vi "UDP - Data System (SubVI).vi"(8 "error in (no error)":errorcluster, 11 "Data":string="\u000204\u0001\u0000ÿ\u0000è\u0003\u0000\u0000\u0000\u0019\u0000\u00002\u0000\u0000\u0000\u001e\u0000\u0000\u0000\u0000\u0000@@\u0000\u0000 @Õ\u0000\u0000\u00002\u0000\u0000\u0000\u0000\u0000€?Ð\u0007\u0000\u0000K") -> (0 "error out":errorcluster, 3 "Data System":T1, 4 "Success":bool)   [LabVIEW 2019]
panel:
  in  "Data 2":string="\u0000\u0000;:\u0000ï²k7ªª5@%\u0019è?\u0000\u0000\u0000\u0000«\u0000\u0000\u0000ÈA\u0000\u0000\u0000\u0000\u000f\u0000\u0000\u0000\u0007\u0000\u0000\u0000Disp\u0000\u0000\u0000\u0000\u0000"
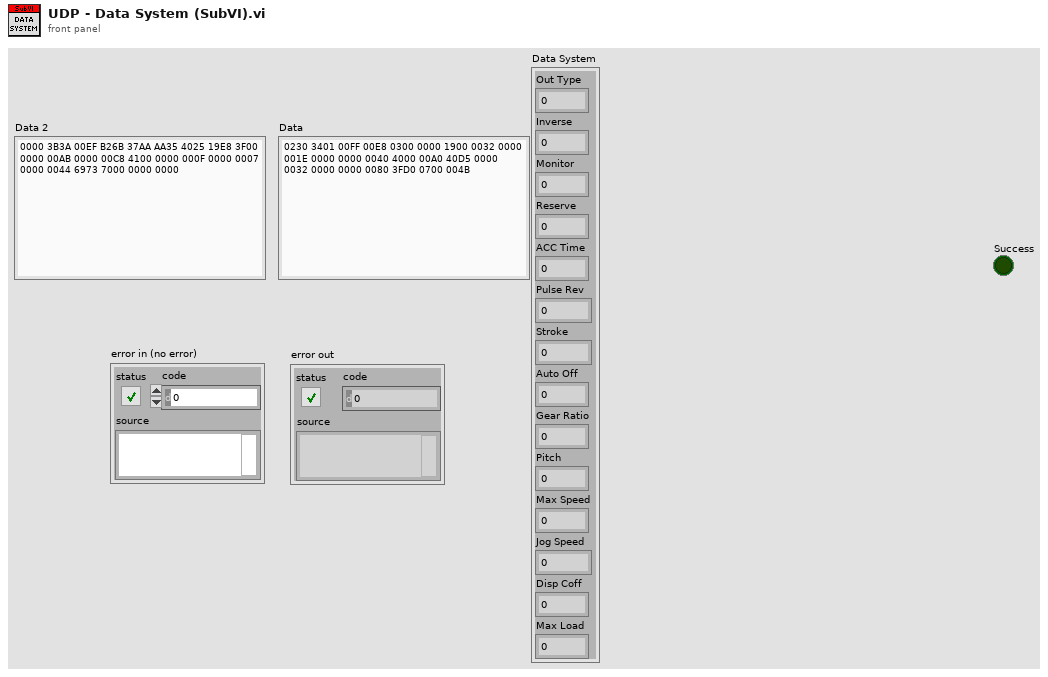
[diagram p1: front panel]
types:
  T1 = cluster{"Out Type":u8, "Inverse":u8, "Monitor":u8, "Reserve":u8, "ACC Time":u32, "Pulse Rev":u32, "Stroke":u32, "Auto Off":u32, "Gear Ratio":sgl, "Pitch":sgl, "Max Speed":u32, "Jog Speed":u32, "Disp Coff":sgl, "Max Load":u32}
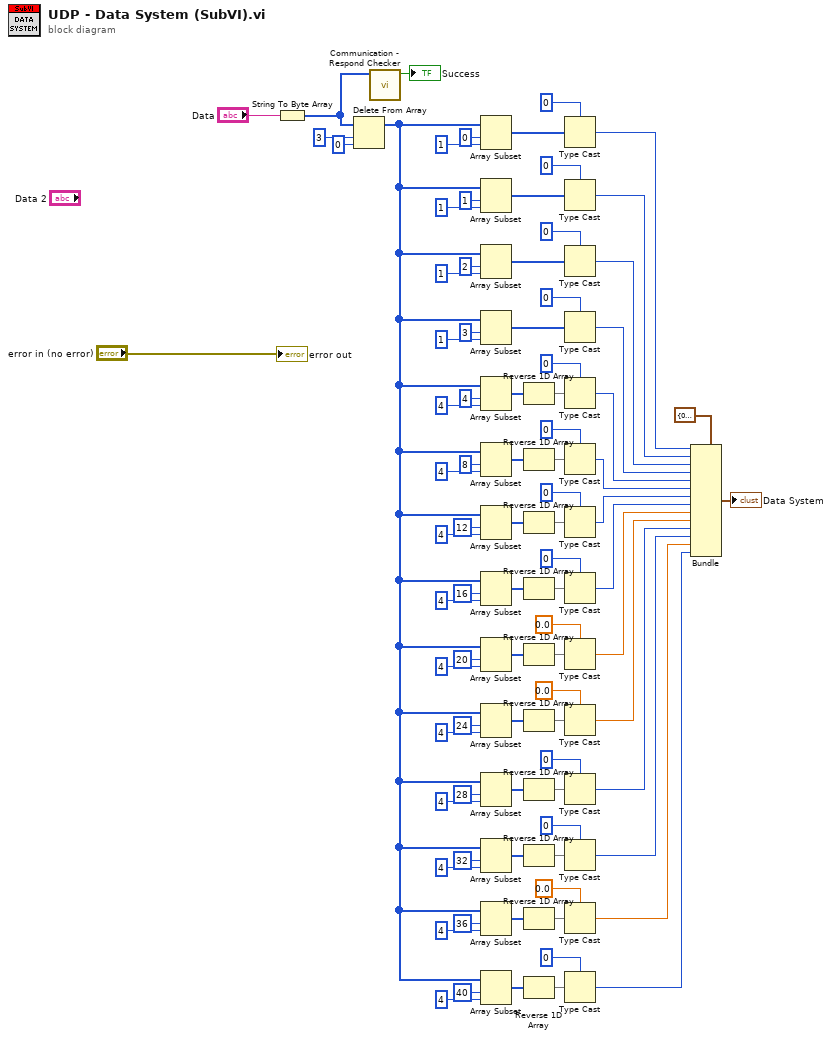
[diagram p0: block diagram]
diagram:
  n1 = String To Byte Array(string="Data") -> (unsigned byte array=w21:u8[])
  n2 = Delete From Array(array=w21, length=3, index=0) -> (array with subset deleted=w5:u8[])  [unwired: 1 out]
  n3 = call "Communication - Respond Checker.vi"("Read Data"=w21) -> ("Success"=→"Success":bool)  [unwired: 10 in]
  n4 = Array Subset(array=w5, index=0, length=1) -> (w20:u8[])
  n5 = Array Subset(array=w5, index=1, length=1) -> (w19:u8[])
  n6 = Array Subset(array=w5, index=2, length=1) -> (w18:u8[])
  n7 = Array Subset(array=w5, index=3, length=1) -> (w17:u8[])
  n8 = Array Subset(array=w5, index=4, length=4) -> (w72:u8[])
  n9 = Array Subset(array=w5, index=8, length=4) -> (w49:u8[])
  n10 = Array Subset(array=w5, index=12, length=4) -> (w54:u8[])
  n11 = Array Subset(array=w5, index=16, length=4) -> (w59:u8[])
  n12 = Array Subset(array=w5, index=20, length=4) -> (w64:u8[])
  n13 = Array Subset(array=w5, index=24, length=4) -> (w38:u8[])
  n14 = Array Subset(array=w5, index=28, length=4) -> (w44:u8[])
  n15 = Array Subset(array=w5, index=32, length=4) -> (w36:u8[])
  n16 = Array Subset(array=w5, index=36, length=4) -> (w14:u8[])
  n17 = Array Subset(array=w5, index=40, length=4) -> (w11:u8[])
  n18 = Reverse 1D Array(array=w72) -> (reversed array=w71:u8[])
  n19 = Reverse 1D Array(array=w49) -> (reversed array=w50:u8[])
  n20 = Reverse 1D Array(array=w54) -> (reversed array=w53:u8[])
  n21 = Reverse 1D Array(array=w59) -> (reversed array=w60:u8[])
  n22 = Reverse 1D Array(array=w64) -> (reversed array=w63:u8[])
  n23 = Reverse 1D Array(array=w38) -> (reversed array=w37:u8[])
  n24 = Reverse 1D Array(array=w44) -> (reversed array=w45:u8[])
  n25 = Reverse 1D Array(array=w36) -> (reversed array=w16:u8[])
  n26 = Reverse 1D Array(array=w14) -> (reversed array=w15:u8[])
  n27 = Reverse 1D Array(array=w11) -> (reversed array=w10:u8[])
  n28 = Type Cast(type=u8 0, x=w20) -> (*(type *) &x=w35:u8)
  n29 = Type Cast(type=u8 0, x=w19) -> (*(type *) &x=w34:u8)
  n30 = Type Cast(type=u8 0, x=w18) -> (*(type *) &x=w33:u8)
  n31 = Type Cast(type=u8 0, x=w17) -> (*(type *) &x=w32:u8)
  n32 = Type Cast(type=u32 0, x=w71) -> (*(type *) &x=w31:u32)
  n33 = Type Cast(type=u32 0, x=w50) -> (*(type *) &x=w30:u32)
  n34 = Type Cast(type=u32 0, x=w53) -> (*(type *) &x=w29:u32)
  n35 = Type Cast(type=u32 0, x=w60) -> (*(type *) &x=w28:u32)
  n36 = Type Cast(type=sgl 0.0, x=w63) -> (*(type *) &x=w27:sgl)
  n37 = Type Cast(type=sgl 0.0, x=w37) -> (*(type *) &x=w26:sgl)
  n38 = Type Cast(type=u32 0, x=w45) -> (*(type *) &x=w25:u32)
  n39 = Type Cast(type=u32 0, x=w16) -> (*(type *) &x=w24:u32)
  n40 = Type Cast(type=sgl 0.0, x=w15) -> (*(type *) &x=w4:sgl)
  n41 = Type Cast(type=u32 0, x=w10) -> (*(type *) &x=w3:u32)
  n42 = Bundle(cluster=T1 {"Out Type"=0, "Inverse"=0, "Monitor"=0, "Reserve"=0, "ACC Time"=0, "Pulse Rev"=0, "Stroke"=0, "Auto Off"=0, "Gear Ratio"=0.0, "Pitch"=0.0, "Max Speed"=0, "Jog Speed"=0, "Disp Coff"=0.0, "Max Load"=0}, "Out Type"=w35, "Inverse"=w34, "Monitor"=w33, "Reserve"=w32, "ACC Time"=w31, "Pulse Rev"=w30, "Stroke"=w29, "Auto Off"=w28, "Gear Ratio"=w27, "Pitch"=w26, "Max Speed"=w25, "Jog Speed"=w24, "Disp Coff"=w4, "Max Load"=w3) -> (→"Data System":T1)
  "error out" <- "error in (no error)"
